vi "Arduino_Serial_FSM.vi"(0 "commands_q":refnum<queue>, 5 "sensor_data_q":refnum<queue>, 11 "error in (no error)":errorcluster) -> (15 "error out":T1)   [LabVIEW 2021, in "GPIB_UART.lvlib"]
uses:
  GPIB_UART.lvlib
  <vilib>/Instr/_visa.llb/VISA Configure Serial Port (Instr).vi
panel:
  in  "VISA resource name out":refnum<visa-resource-name>
  in  "Power ON | OFF":bool
  out "Sampling Frequency":string="1"
  out "baud RATE":string="9600"
  out "COM port":string="COM5"
  out "Waveform Graph":dbl[](graph)
  in  "Arguments":string
  in  "state_and_args":string
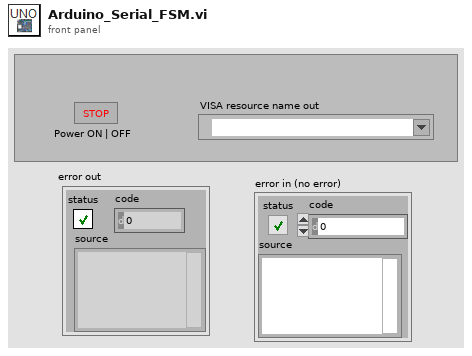
[diagram p1: front panel]
types:
  T1 = cluster{"status":bool, "code":u8, "source":string}
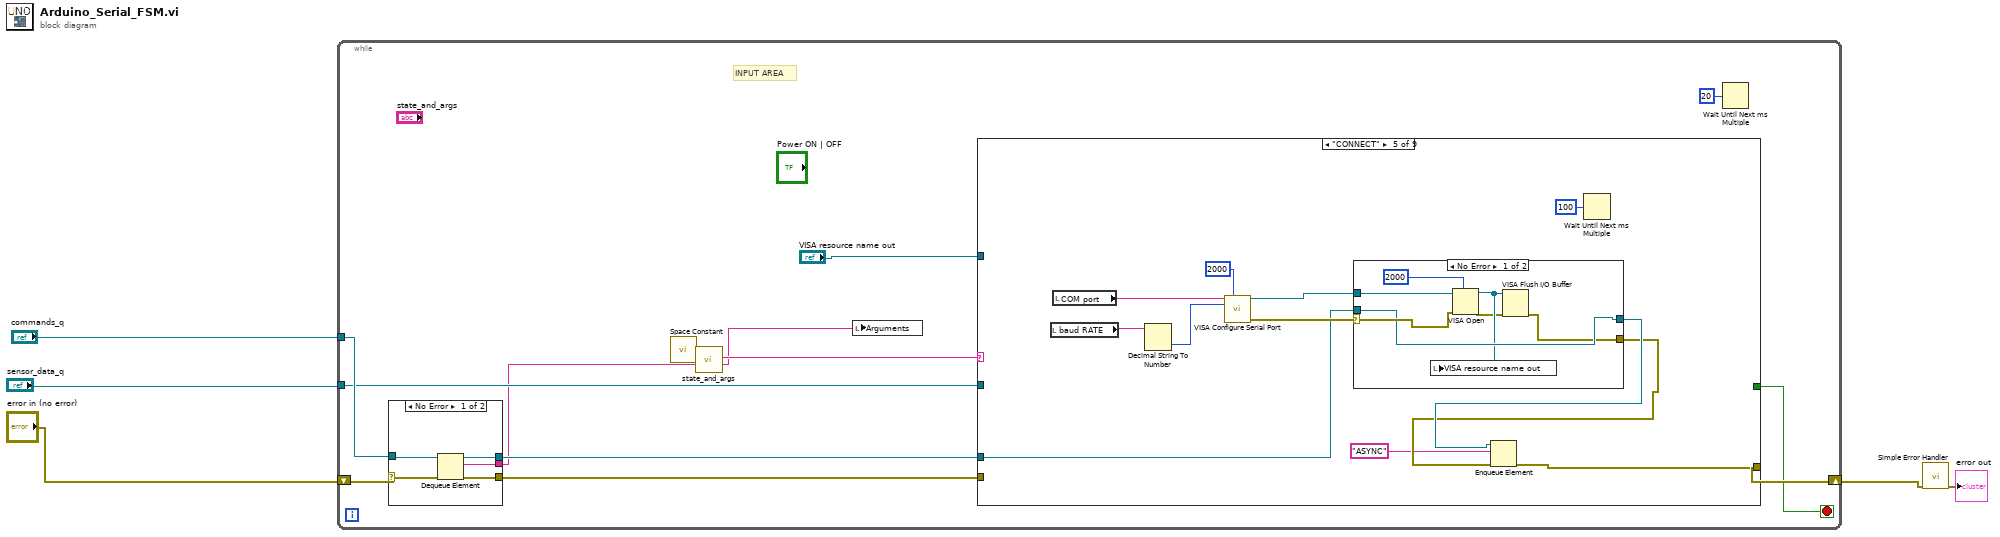
[diagram p0: block diagram]
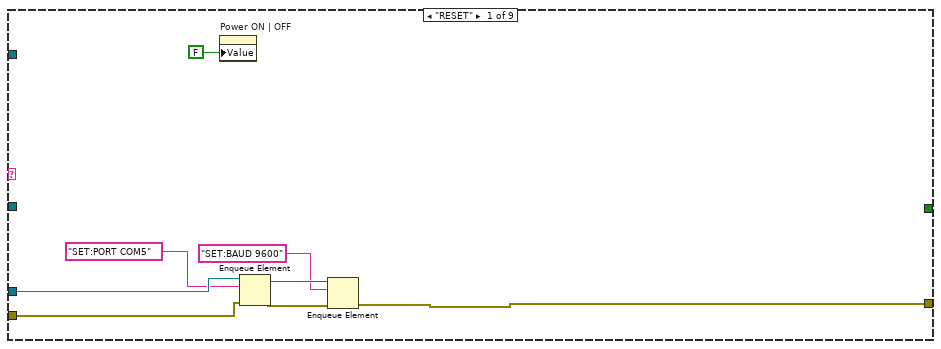
[diagram p2: hidden frame]
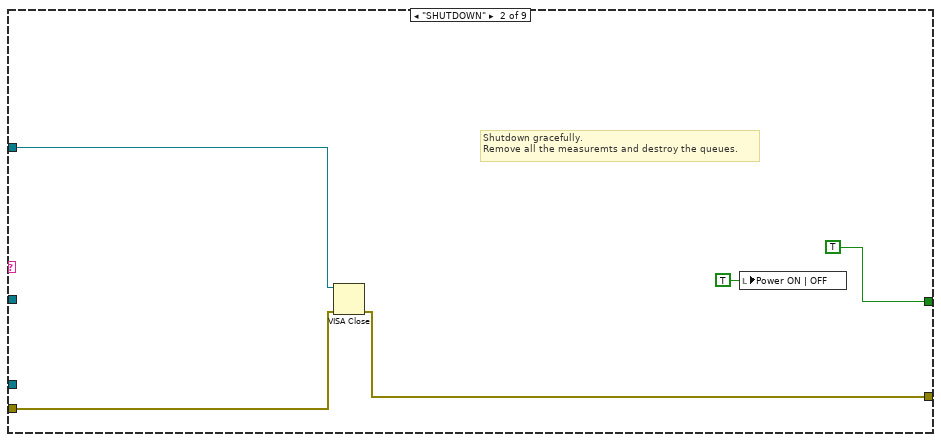
[diagram p3: hidden frame]
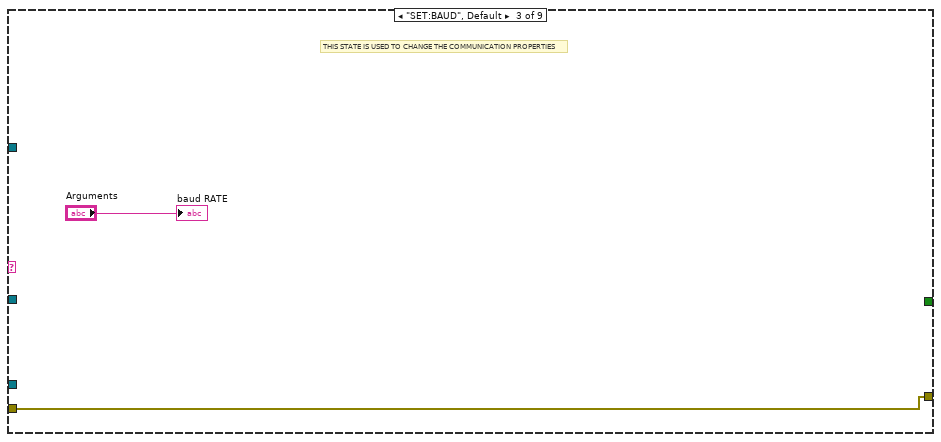
[diagram p4: hidden frame]
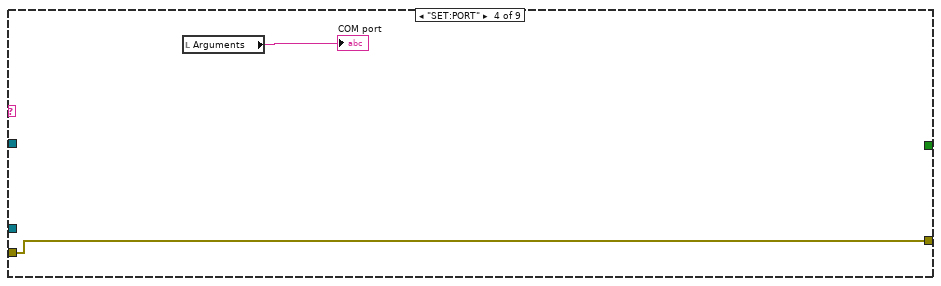
[diagram p5: hidden frame]
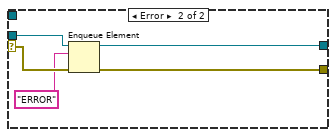
[diagram p6: hidden frame]
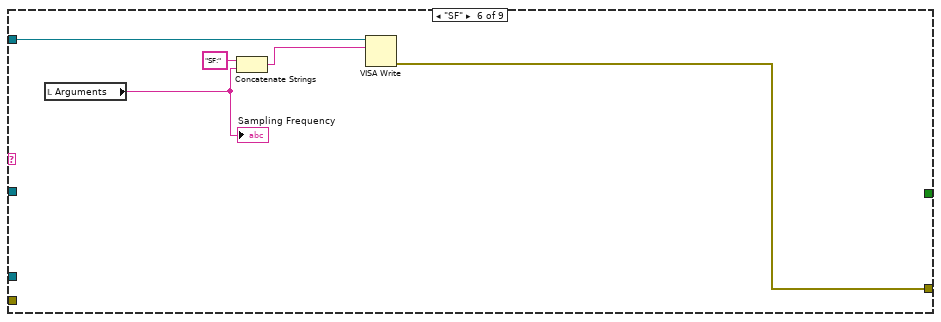
[diagram p7: hidden frame]
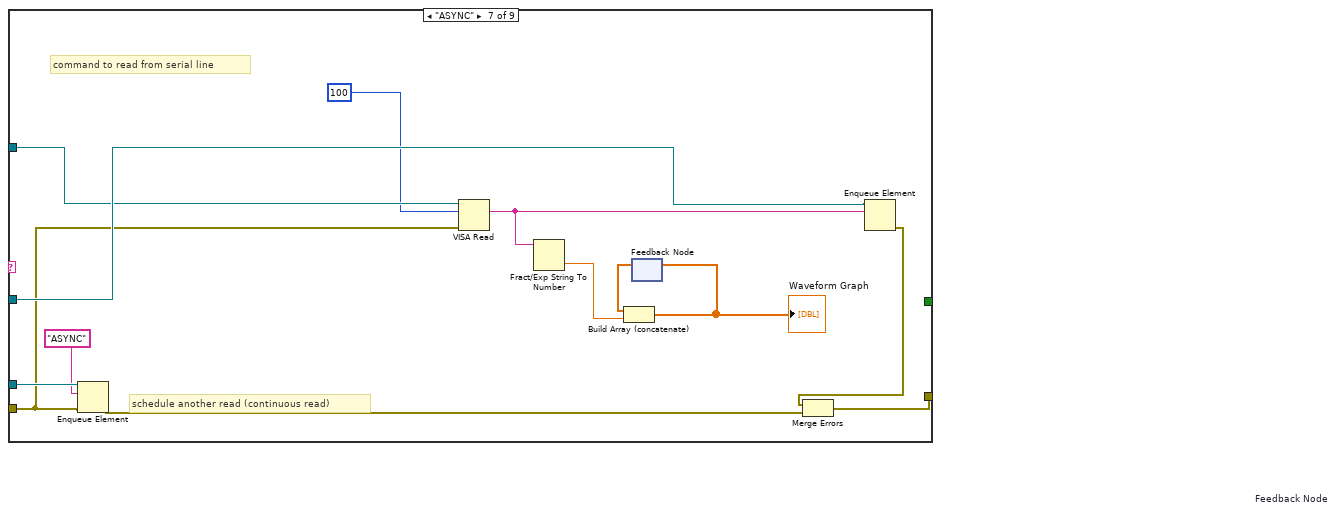
[diagram p8: hidden frame]
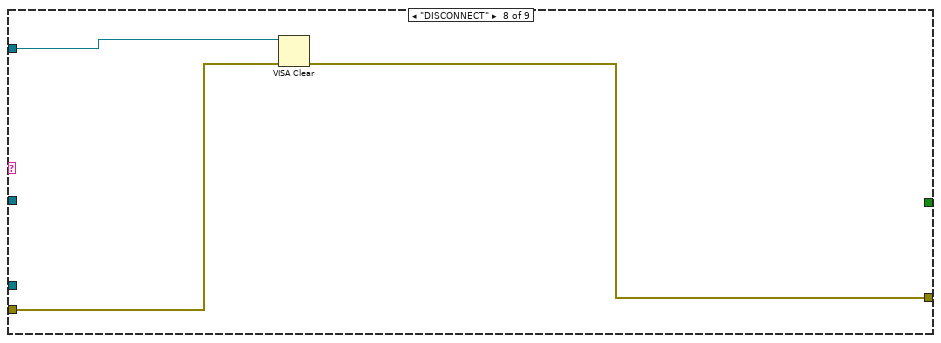
[diagram p9: hidden frame]
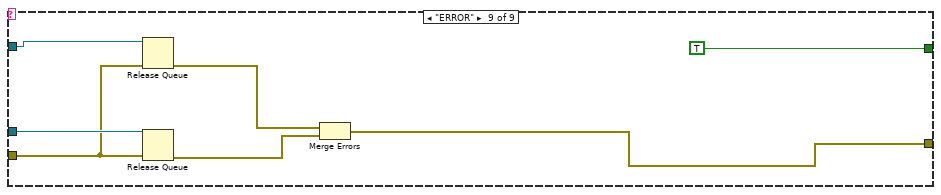
[diagram p10: hidden frame]
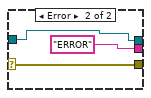
[diagram p11: hidden frame]
diagram:
  n1 = while {
    tunnel: "commands_q" -> [w17]
    shift-right: [w14] -> w4
    shift-left: "error in (no error)" -> [w18]
    tunnel: "sensor_data_q" -> [w13]
    stop <- w12 stop-if-true
    # "INPUT AREA"
    n2 = case shown="No Error" w18 {
      selector: w18 -> [w92 w93]
      tunnel: w17 -> [w91 w94]
      tunnel: [w90 w94] -> w16
      tunnel: [w89 w93] -> w15
      tunnel: [w88 "ERROR"] -> w9
      frame No Error {
        n3 = Dequeue Element(queue=w91, error in (no error)=w92) -> (queue out=w90:refnum<queue>, element=w88:string, error out=w89:errorcluster)  [unwired: 1 in, 1 out]
      }
      frame Error {
      }
    }
    n4 = call <vilib>:"Space Constant.vi"() -> ("String"=w8:string)
    n5 = call "state_and_args.vi"("String"=w9, "DELIMITER (:)"=w8) -> ("Arguments"=w6:string, "State"=w7:string)  [unwired: 8 in]
    n6 = local write "Arguments"(w6) -> ()
    n7 = case shown="\"CONNECT\"" w7 {
      tunnel: w16 -> [w25 _ _ _ w41 _ w77 _ w86]
      tunnel: w15 -> [w20 w28 w32 w34 _ _ w70 w80 w85]
      tunnel: [w19 w27 w32 w34 w37 w62 w75 w79 w82] -> w14
      tunnel: w13 -> [_ _ _ _ _ _ w73 _ w87]
      tunnel: [_ TRUE _ _ _ _ _ _ TRUE] -> w12
      tunnel: "VISA resource name out" -> [_ w29 _ _ _ w61 w71 w78 _]
      frame "RESET" {
        n8 = property on="Power ON | OFF" class="Bool (strict)"("Value"=FALSE ("Blinking")) -> ()  [unwired: 2 in, 2 out]
        n9 = Enqueue Element(queue=w25, element="SET:PORT COM5", error in (no error)=w20) -> (queue out=w23:refnum<queue>, error out=w22:errorcluster)  [unwired: 1 in, 1 out]
        n10 = Enqueue Element(queue=w23, element="SET:BAUD 9600", error in (no error)=w22) -> (error out=w19:errorcluster)  [unwired: 1 in, 2 out]
      }
      frame "SHUTDOWN" {
        # "Shutdown gracefully.\nRemove all the measuremts and destroy the queues."
        n11 = VISA Close(VISA resource name=w29, error in (no error)=w28) -> (error out=w27:errorcluster)
        n12 = local write "Power ON | OFF"(TRUE ("Power ON | OFF")) -> ()
      }
      frame "SET:BAUD", Default {
        # "THIS STATE IS USED TO CHANGE THE COMMUNICATION PROPERTIES"
        "baud RATE" <- "Arguments"
      }
      frame "SET:PORT" {
        n13 = local read "Arguments"() -> (→"COM port":string)
      }
      frame "CONNECT" {
        n14 = local read "baud RATE"() -> (w46:string)
        n15 = local read "COM port"() -> (w47:string)
        n16 = Decimal String To Number(string=w46) -> (number=w45:i32)  [unwired: 2 in, 1 out]
        n17 = call-poly "VISA Configure Serial Port"("VISA resource name"=w47, "timeout (10sec)"=u32 2000, "baud rate (9600)"=w45) -> ("VISA resource name out"=w43:refnum<visa-resource-name>, "error out"=w42:errorcluster)  [unwired: 11 in]
        n18 = case shown="No Error" w42 {
          selector: w42 -> [w53 w59]
          tunnel: w43 -> [w54 _]
          tunnel: w41 -> [w51 w58]
          tunnel: [w50 w56] -> w39
          tunnel: [w51 w55] -> w40
          frame No Error {
            n19 = VISA Open(timeout (0)=u32 2000 ("VISA Open timeout (0)"), error in (no error)=w53, VISA resource name=w54) -> (VISA resource name=w49:refnum<visa-resource-name>, error out=w48:errorcluster)  [unwired: 2 in]
            n20 = local write "VISA resource name out"(w49) -> ()
            n21 = VISA Flush I/O Buffer(VISA resource name=w49, error in (no error)=w48) -> (error out=w50:errorcluster)  [unwired: 1 in, 1 out]
          }
          frame Error {
            n22 = Enqueue Element(queue=w58, element="ERROR", error in (no error)=w59) -> (queue out=w55:refnum<queue>, error out=w56:errorcluster)  [unwired: 1 in, 1 out]
          }
        }
        n23 = Enqueue Element(queue=w40, element="ASYNC", error in (no error)=w39) -> (error out=w37:errorcluster)  [unwired: 1 in, 2 out]
        n24 = Wait Until Next ms Multiple(millisecond multiple=u32 100) -> ()  [unwired: 1 out]
      }
      frame "SF" {
        n25 = local read "Arguments"() -> (w60:string)
        "Sampling Frequency" <- w60
        n26 = Concatenate Strings("SF:" ("string"), w60) -> (w63:string)
        n27 = VISA Write(VISA resource name=w61, write buffer=w63) -> (error out=w62:errorcluster)  [unwired: 1 in, 2 out]
      }
      frame "ASYNC" {
        # "command to read from serial line"
        # "schedule another read (continuous read)"
        n28 = Enqueue Element(queue=w77, element="ASYNC", error in (no error)=w70) -> (error out=w74:errorcluster)  [unwired: 1 in, 2 out]
        n29 = VISA Read(VISA resource name=w71, byte count=u32 100, error in (no error)=w70) -> (read buffer=w65:string)  [unwired: 3 out]
        n30 = Fract/Exp String To Number(string=w65) -> (number=w66:dbl)  [unwired: 3 in, 1 out]
        n31 = feedback #1 "Feedback Node"() -> (w68:dbl[])  [unwired: 1 in]
        n32 = Build Array (concatenate)(w68, w66) -> (w67:dbl[])
        "Waveform Graph" <- w67
        n33 = feedback-in #1(w67) -> ()
        n34 = Enqueue Element(queue=w73, element=w65) -> (error out=w72:errorcluster)  [unwired: 2 in, 2 out]
        n35 = Merge Errors(w72, w74) -> (w75:errorcluster)
      }
      frame "DISCONNECT" {
        n36 = VISA Clear(VISA resource name=w78, error in (no error)=w80) -> (error out=w79:errorcluster)  [unwired: 1 out]
      }
      frame "ERROR" {
        n37 = Release Queue(queue=w87, error in (no error)=w85) -> (error out=w84:errorcluster)  [unwired: 1 in, 2 out]
        n38 = Release Queue(queue=w86, error in (no error)=w85) -> (error out=w83:errorcluster)  [unwired: 1 in, 2 out]
        n39 = Merge Errors(w84, w83) -> (w82:errorcluster)
      }
    }
    n40 = Wait Until Next ms Multiple(millisecond multiple=u32 20) -> ()  [unwired: 1 out]
  }
  n41 = call <vilib>:"Simple Error Handler.vi"("error in (no error)"=w4) -> ("error out"=→"error out":errorcluster)  [unwired: 4 in, 4 out]
